vi "OP300ZP_INIT_ST5520.vi"(8 "errin":errorcluster caption="entrée d'erreur (pas d'erreur)", 11 "VISA":refnum<visa-resource-name>) -> (0 "errout":errorcluster caption="sortie d'erreur", 3 "VISA":refnum<visa-resource-name>)   [LabVIEW 2020]
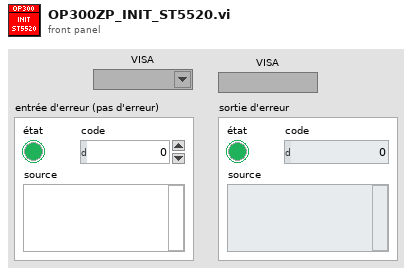
[diagram p1: front panel]
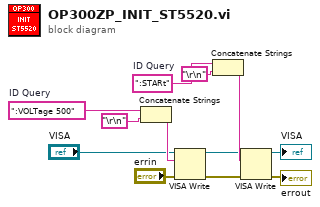
[diagram p0: block diagram]
diagram:
  w10 = ":VOLTage 500"  # ID Query
  w11 = ":STARt"  # ID Query
  n1 = Concatenate Strings(w10, "\r\n") -> (w9:string)
  n2 = VISA Write(VISA resource name="VISA", write buffer=w9, error in (no error)="errin") -> (VISA resource name out=w7:refnum<visa-resource-name>, error out=w1:errorcluster)  [unwired: 1 out]
  n3 = Concatenate Strings(w11, "\r\n") -> (w12:string)
  n4 = VISA Write(VISA resource name=w7, write buffer=w12, error in (no error)=w1) -> (VISA resource name out=→"VISA":refnum<visa-resource-name>, error out=→"errout":errorcluster)  [unwired: 1 out]
